vi "KE622x -- Get Display Params.vi"(0 "Resource In":refnum<visa-resource-name>, 1 "Check For SCPI Errors? (T)":bool=TRUE, 11 "error in (no error)":errorcluster) -> (4 "Resource Out (dupl)":refnum<visa-resource-name>, 8 "Display Params":T1={"Display\nEnabled?"=TRUE, "Custom Top\nLine Text?"=FALSE, "Top Line Text (20 chars max)"="", "Custom Bottom\nLine Text?"=FALSE, "Bottom Line Text (32 chars max)"=""}, 15 "error out":errorcluster)   [LabVIEW 2020, in "Keithley 622x.lvlib"]
doc: "Returns the current set of parameters for the KE622x front panel display."
uses:
  Keithley 622x.lvlib
  Typedefs/KE622x -- Display Params.ctl
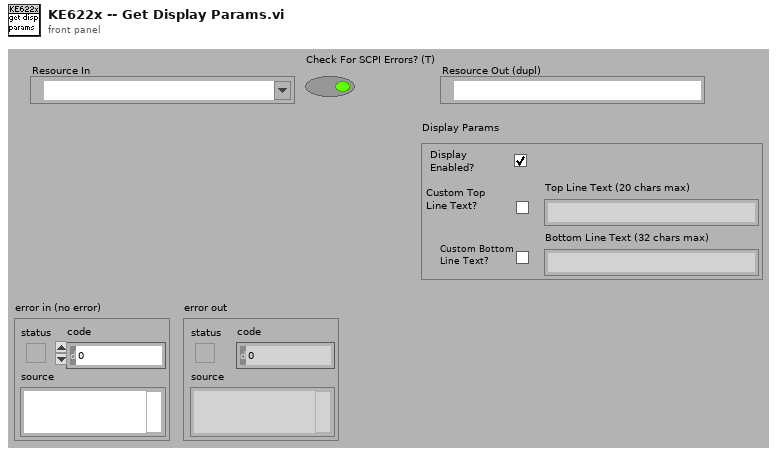
[diagram p1: front panel]
types:
  T1 = typedef "Keithley 622x.lvlib/KE622x -- Display Params.ctl" = cluster{"Display\nEnabled?":bool, "Custom Top\nLine Text?":bool, "Top Line Text (20 chars max)":string, "Custom Bottom\nLine Text?":bool, "Bottom Line Text (32 chars max)":string}
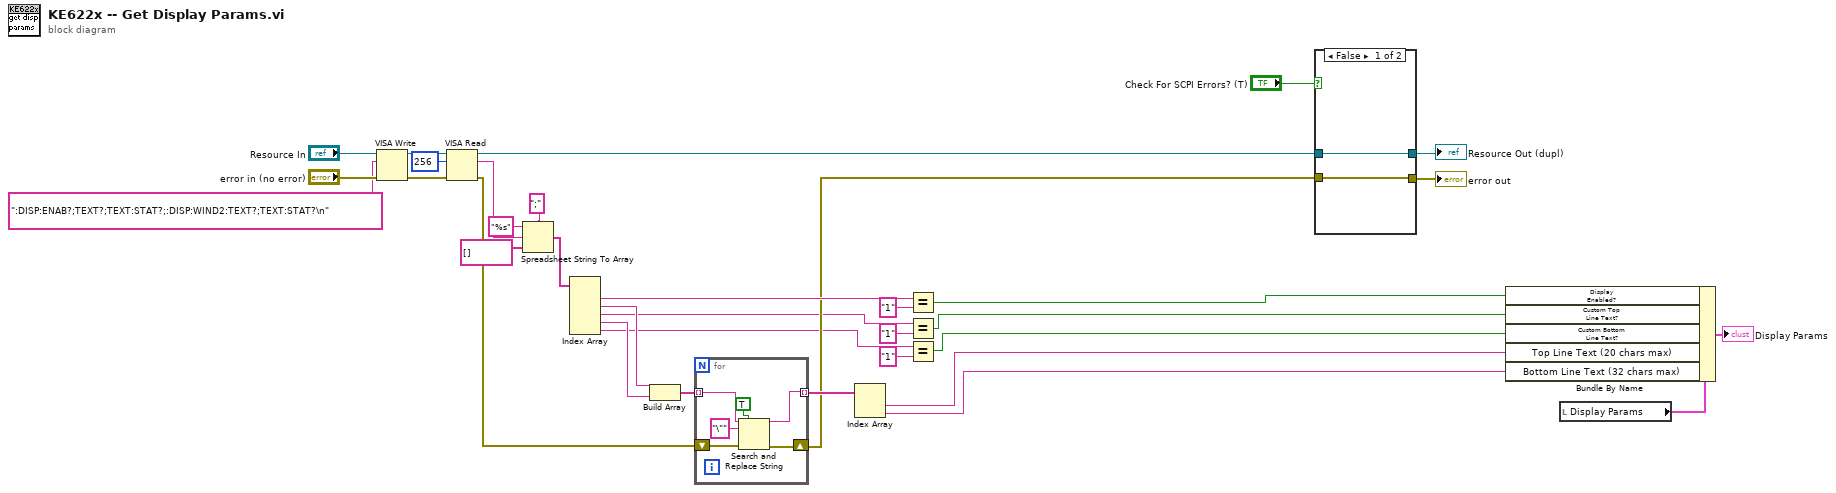
[diagram p0: block diagram]
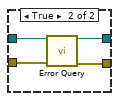
[diagram p2: hidden frame]
diagram:
  n1 = VISA Write(VISA resource name="Resource In", write buffer=":DISP:ENAB?;TEXT?;TEXT:STAT?;:DISP:WIND2:TEXT?;TEXT:STAT?\n" ("format string"), error in (no error)="error in (no error)") -> (VISA resource name out=w28:refnum<visa-resource-name>, error out=w27:errorcluster)  [unwired: 1 out]
  n2 = VISA Read(VISA resource name=w28, byte count=u32 256, error in (no error)=w27) -> (VISA resource name out=w25:refnum<visa-resource-name>, read buffer=w24:string, error out=w13:errorcluster)  [unwired: 1 out]
  n3 = Spreadsheet String To Array(delimiter (Tab)=";", format string="%s", spreadsheet string=w24, array type (2D Dbl)=string[] []) -> (array=w20:string[])
  n4 = Index Array(array=w20) -> (element #1=w19:string, element #2=w6:string, element #3=w5:string, element #4=w4:string, element #5=w3:string)  [unwired: 5 in]
  n5 = Build Array(w6, w4) -> (w14:string[])
  n6 = for {
    tunnel: w14 -> [w37] mode=indexing
    shift-right: [w35] -> w8
    shift-left: w13 -> [w38]
    tunnel: [w36] -> w12 mode=indexing
    n7 = Search and Replace String(replace all?=TRUE ("replace all? (F)"), input string=w37, search string="\"", error in=w38) -> (result string=w36:string, error out=w35:errorcluster)  [unwired: 4 in, 2 out]
  }
  n8 = Index Array(array=w12) -> (element #1=w2:string, element #2=w1:string)  [unwired: 2 in]
  n9 = Equal?(x=w19, y="1") -> (x = y?=w15:bool)
  n10 = Equal?(x=w5, y="1") -> (x = y?=w10:bool)
  n11 = Equal?(x=w3, y="1") -> (x = y?=w9:bool)
  n12 = case shown="False" "Check For SCPI Errors? (T)" {
    tunnel: w25 -> [w42 w46]
    tunnel: w8 -> [w41 w45]
    tunnel: [w41 w44] -> w30
    tunnel: [w42 w43] -> w31
    frame False {
    }
    frame True {
      n13 = call "Error Query.vi"("VISA Resource In"=w46, "error in (no error)"=w45) -> ("VISA Resource Out (dupl)"=w43:refnum<visa-resource-name>, "error out"=w44:errorcluster)  [unwired: 10 in, 2 out]
    }
  }
  "Resource Out (dupl)" <- w31
  "error out" <- w30
  n14 = local read "Display Params"() -> (w16:T1)
  n15 = Bundle By Name(cluster=w16, "Display\nEnabled?"=w15, "Custom Top\nLine Text?"=w10, "Custom Bottom\nLine Text?"=w9, "Top Line Text (20 chars max)"=w2, "Bottom Line Text (32 chars max)"=w1) -> (→"Display Params":T1)
